vi "Add Incoming Section.vi"(7 "highlight? (F)":bool, 8 "error in":errorcluster, 11 "configuration files ref":T1 format="%.0x") -> (0 "error out":errorcluster, 2 "Incoming ref":T1 format="%.0x", 3 "configuration files ref out":T1 format="%.0x")   [LabVIEW 2020, in "Ballard ARINC 429 Scripting.lvlib"]
uses:
  Ballard ARINC 429 Scripting.lvlib
  <vilib>/NI VeriStand/Custom Device API/Custom Device Item Ref.ctl
  Constants.vi
  <vilib>/NI VeriStand/Custom Device Tools/Custom Device Utility Library/NI VeriStand - Search for Item by GUID.vi
  <vilib>/NI VeriStand/Custom Device API/Custom Device API.lvlib
  <vilib>/NI VeriStand/Custom Device Tools/Custom Device Utility Library/Custom Device Utility Library.lvlib
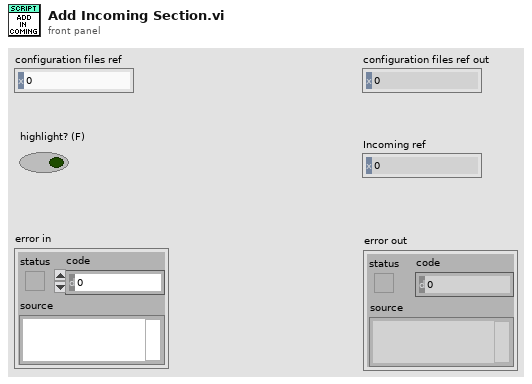
[diagram p1: front panel]
types:
  T1 = typedef "Custom Device API.lvlib/Custom Device Item Ref.ctl" = u64
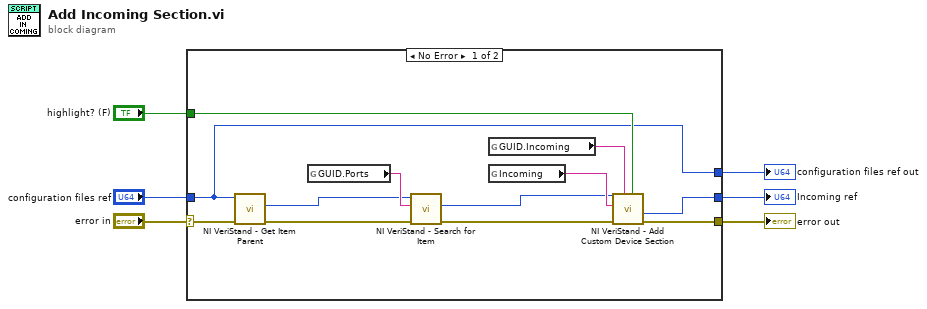
[diagram p0: block diagram]
diagram:
  n1 = case shown="No Error" "error in" {
    selector: "error in" -> [w11 w20]
    tunnel: "highlight? (F)" -> [w17 _]
    tunnel: "configuration files ref" -> [w7 w19]
    tunnel: [w16 w20] -> w4
    tunnel: [w8 _] -> w3
    tunnel: [w7 w19] -> w1
    frame No Error {
      n2 = call <vilib>:"NI VeriStand - Get Item Parent.vi"("error in (no error)"=w11, "Item Ref in"=w7) -> ("error out"=w10:errorcluster, "Parent Ref"=w9:T1)  [unwired: 6 in, 2 out]
      n3 = global read "Constants.vi" "GUID.Ports"() -> (w14:string)
      n4 = call-poly <vilib>:"NI VeriStand - Search for Item.vi"("error in"=w10, "Item GUID"=w14, "Section Ref in"=w9) -> ("error out"=w13:errorcluster, "Item Ref"=w12:T1)  [unwired: 5 in, 2 out]
      n5 = global read "Constants.vi" "GUID.Incoming"() -> (w18:string)
      n6 = global read "Constants.vi" "Incoming"() -> (w15:string)
      n7 = call <vilib>:"NI VeriStand - Add Custom Device Section.vi"("Highlight? (F)"=w17, "GUID (Default Section)"=w18, "error in (no error)"=w13, "Section Name"=w15, "Parent Ref in"=w12) -> ("error out"=w16:errorcluster, "Section Ptr"=w8:T1)  [unwired: 3 in, 2 out]
    }
    frame Error {
    }
  }
  "error out" <- w4
  "Incoming ref" <- w3
  "configuration files ref out" <- w1
